vi "STP_Engine_Main.vi"(6 "Log Data?":bool, 8 "error in":errorcluster, 9 "notifier in":refnum<notifier>, 10 "Socket No":i16, 11 "Selected Sockets":i16[](array[numeric])) -> (0 "error out":errorcluster)   [LabVIEW 2023, in "HardwareAbstractionLayer_LVOOP.lvlib" / "CAN Application Protocols Lib.lvlib" / "STP Protocol.lvclass"]
uses:
  STP Protocol.lvclass
  Ctrls/STP Output Data.ctl
  Ctrls/STP Error Cluster.ctl
  Teststand Steptypes/CAN/CAN Engine/Control/CAN FGV State.ctl
  <vilib>/xnet/xnet.llb/XNET Frame CAN.ctl
  <vilib>/xnet/xnet.llb/XNET Frame Type CAN.ctl
  Ctrls/STP States.ctl
  Ctrls/STP Engine States.ctl
  Teststand Steptypes/CAN/CAN Engine/STP Engine SubVI/Control/STP Engine Rx Data.ctl
  Ctrls/STP Loop Data.ctl
  STP Protocol.lvclass/STP Protocol.ctl
  Ctrls/TP Frame Type.ctl
  0913cad6-f2c8-4594-8002-bcfba81b39ef.vi
  d64f42c0-1e64-4e1b-9106-5438a7ab598d.vi
  ddd6aa9f-f484-4e89-88b8-35a021554d50.vi
  7032564a-a6a9-40e0-a5d6-1f35f757e68a.vi
  Teststand Steptypes/LTT_TeststandSteptypes.lvlib
panel:
  out "RequestTimeout?":bool
  out "STP Output Data":T1
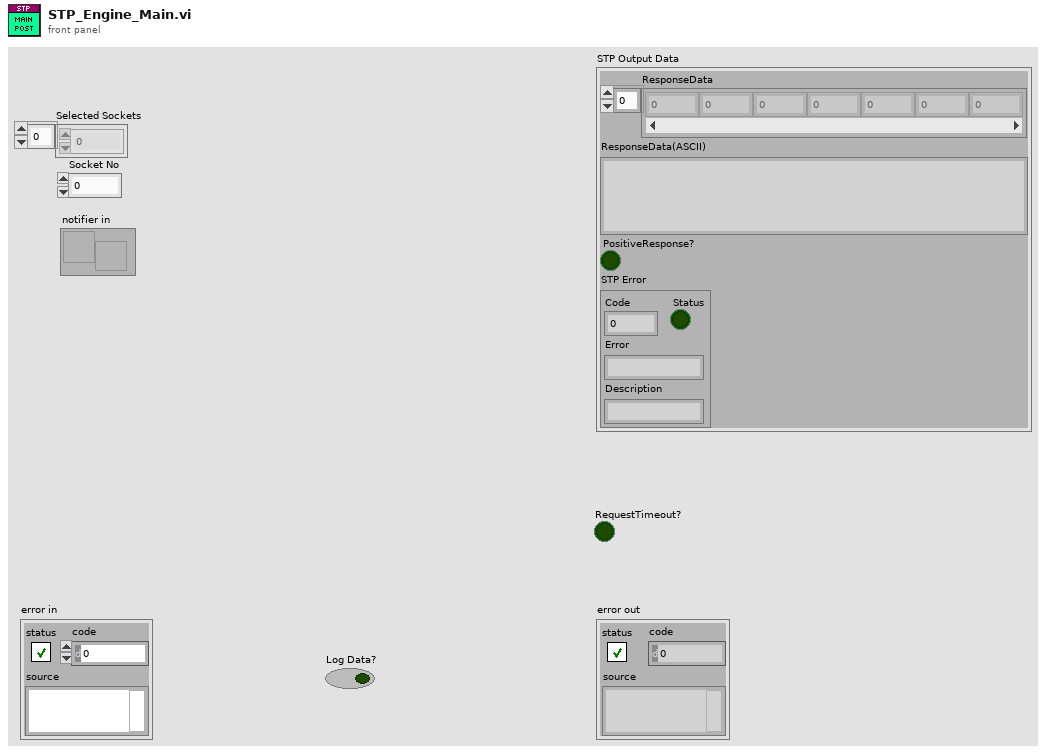
[diagram p1: front panel]
types:
  T1 = typedef "HardwareAbstractionLayer_LVOOP.lvlib/CAN Application Protocols Lib.lvlib/STP Protocol.lvclass/STP Output Data.ctl" = cluster{"ResponseData":u8[], "ResponseData(ASCII)":string, "PositiveResponse?":bool, "STP Error":T2}
  T2 = typedef "HardwareAbstractionLayer_LVOOP.lvlib/CAN Application Protocols Lib.lvlib/STP Protocol.lvclass/STP Error Cluster.ctl" = cluster{"Status":bool, "Code":u8, "Error":string, "Description":string}
  T3 = typedef "XNET Frame CAN.ctl" = cluster{"timestamp":timestamp, "payload":u8[], "identifier":u32, "type":T4, "extended?":bool, "echo?":bool}
  T4 = typedef "XNET Frame Type CAN.ctl" = u8
  T5 = typedef "LTT_TeststandSteptypes.lvlib/CAN FGV State.ctl" = enum16{"Init", "Get", "Set"}
  T6 = typedef "HardwareAbstractionLayer_LVOOP.lvlib/CAN Application Protocols Lib.lvlib/STP Protocol.lvclass/STP Engine States.ctl" = enum16{"Idle", "Poll", "Run"}
  T7 = typedef "HardwareAbstractionLayer_LVOOP.lvlib/CAN Application Protocols Lib.lvlib/STP Protocol.lvclass/STP States.ctl" = enum16{"Init", "Send Request", "Check Ack", "Send TP Frames", "Send Flow Control Frame", "Check Response", "Read TP Data", "Return Data", "Return Positive Response", "Return Error Response", "Exit"}
  T8 = typedef "LTT_TeststandSteptypes.lvlib/STP Engine Rx Data.ctl" = cluster{"STP Output Data":T1, "RequestTimeout?":bool}
  T9 = typedef "HardwareAbstractionLayer_LVOOP.lvlib/CAN Application Protocols Lib.lvlib/STP Protocol.lvclass/STP Loop Data.ctl" = cluster{"ResponseData":u8[], "DataSize(bytes)":u16, "ReceiveAllData?":bool, "PositiveResponse?":bool, "CosecutiveFrameID":fxp<+,4,4>, "#FrameToRead":i32}
  T10 = typedef "LTT_TeststandSteptypes.lvlib/STP Engine Tx Data.ctl" = cluster{"STP Input Data":T11, "Socket No":u16}
  T11 = typedef "HardwareAbstractionLayer_LVOOP.lvlib/CAN Application Protocols Lib.lvlib/STP Protocol.lvclass/STP Input Data.ctl" = cluster{"TxID":u32, "RxID":u32, "CMD":T12, "RQ Data":u8[], "+veResponseCode":u8, "ResponseTimeout (S)":dbl}
  T12 = typedef "HardwareAbstractionLayer_LVOOP.lvlib/CAN Application Protocols Lib.lvlib/STP Protocol.lvclass/STP CMD.ctl" = u8
  T13 = typedef "HardwareAbstractionLayer_LVOOP.lvlib/CAN Application Protocols Lib.lvlib/STP Protocol.lvclass/TP Frame Type.ctl" = u8
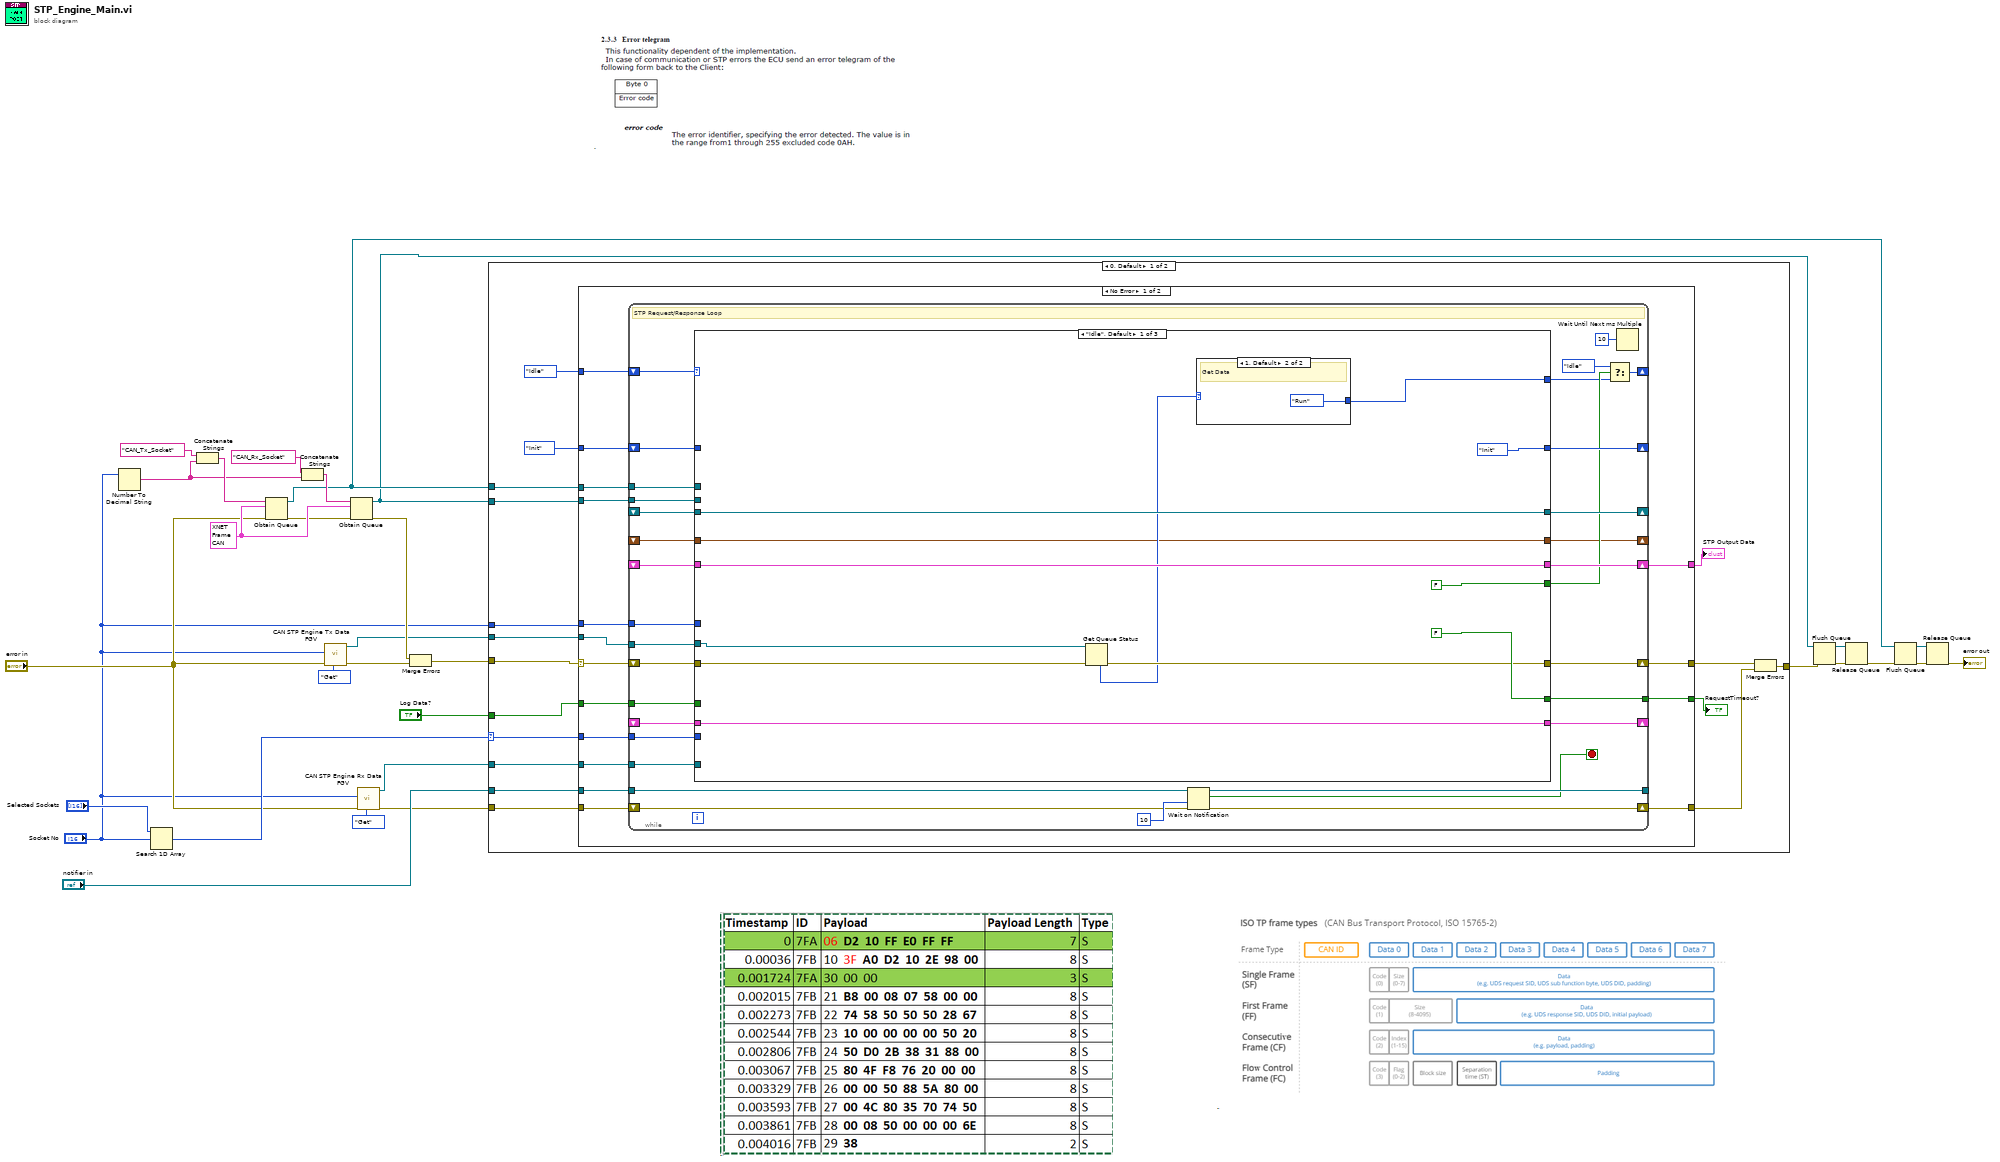
[diagram p0: block diagram]
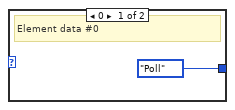
[diagram p2: hidden frame]
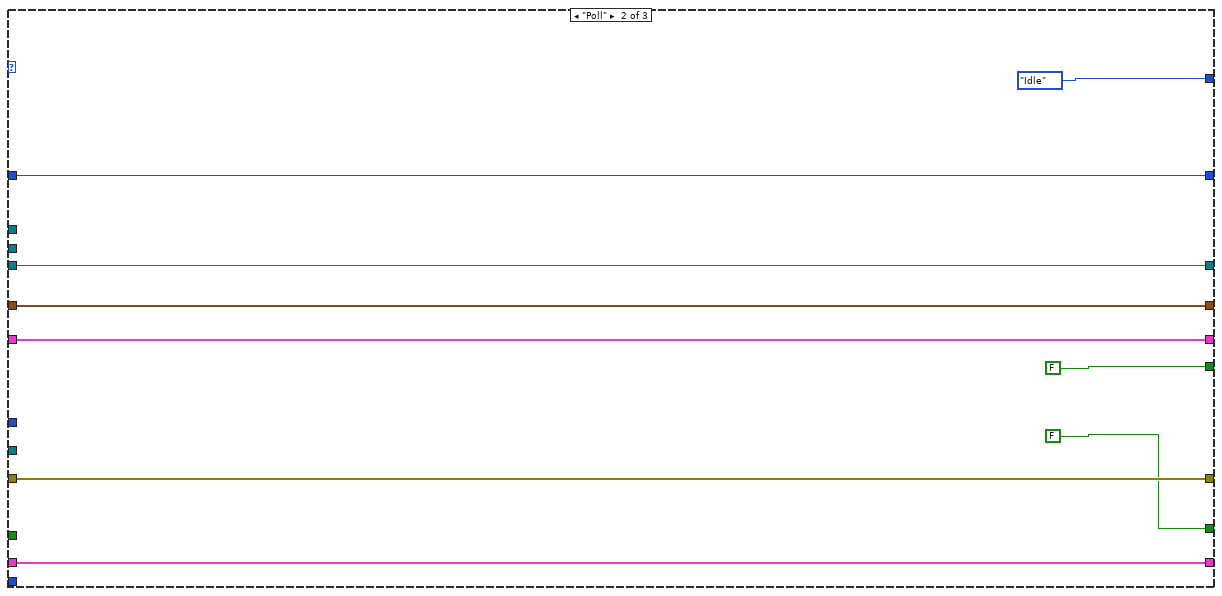
[diagram p3: hidden frame]
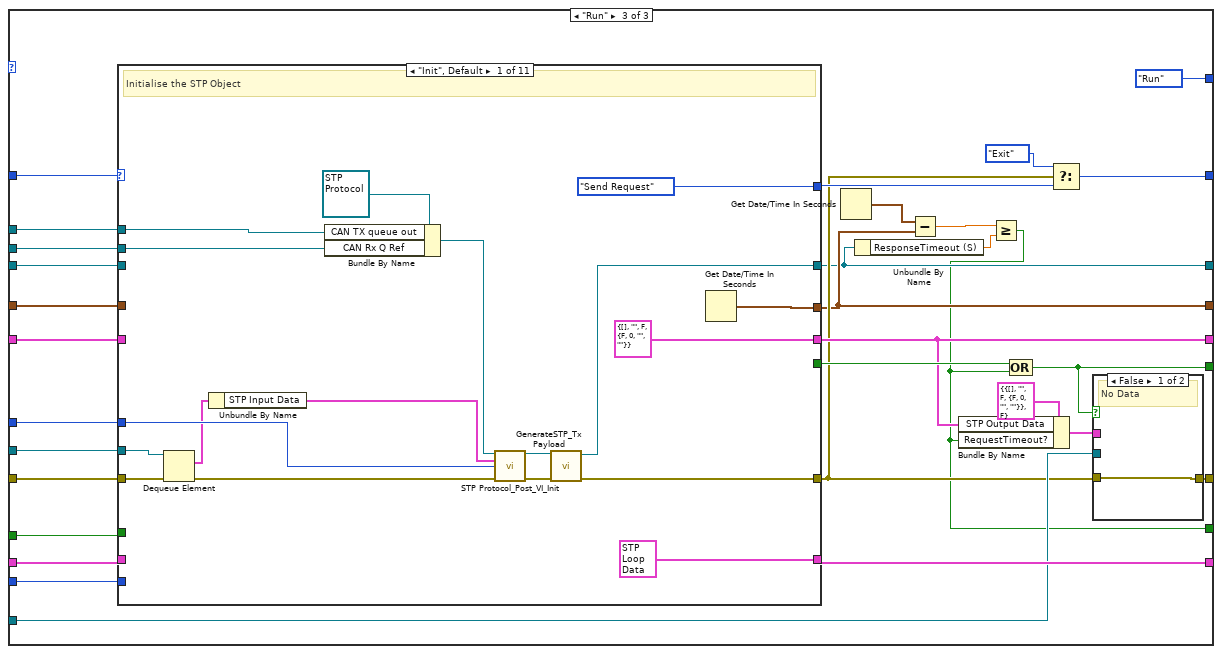
[diagram p4: hidden frame]
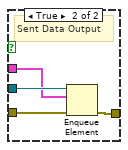
[diagram p5: hidden frame]
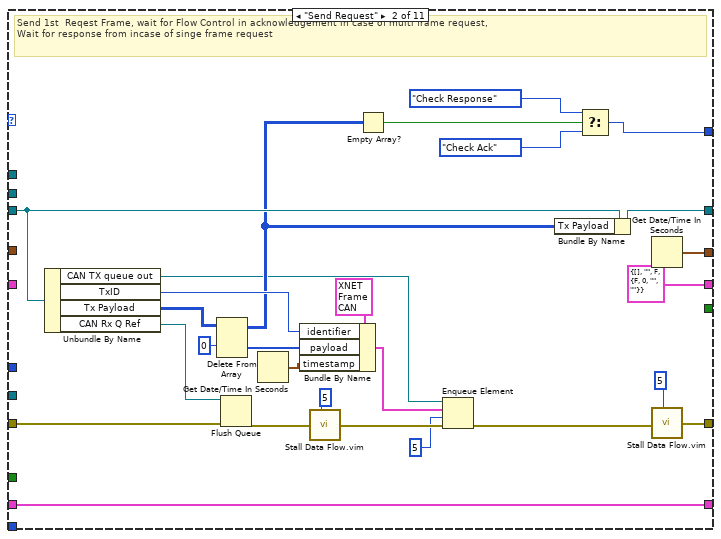
[diagram p6: hidden frame]
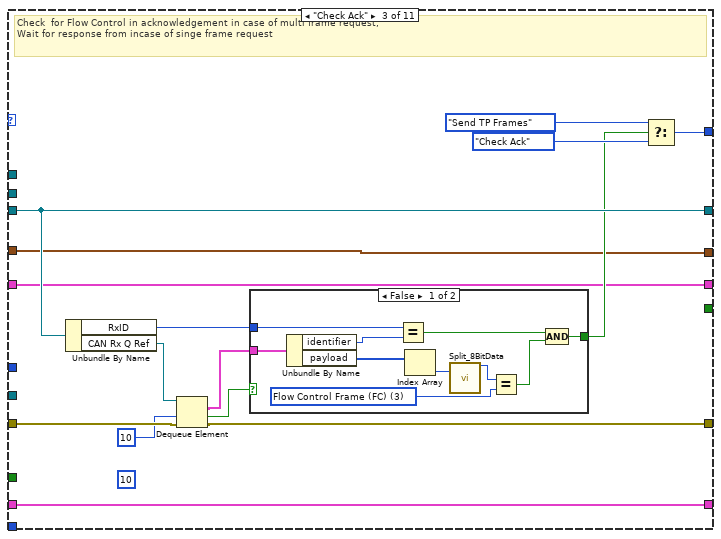
[diagram p7: hidden frame]
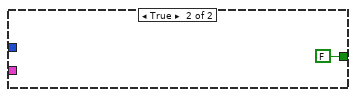
[diagram p8: hidden frame]
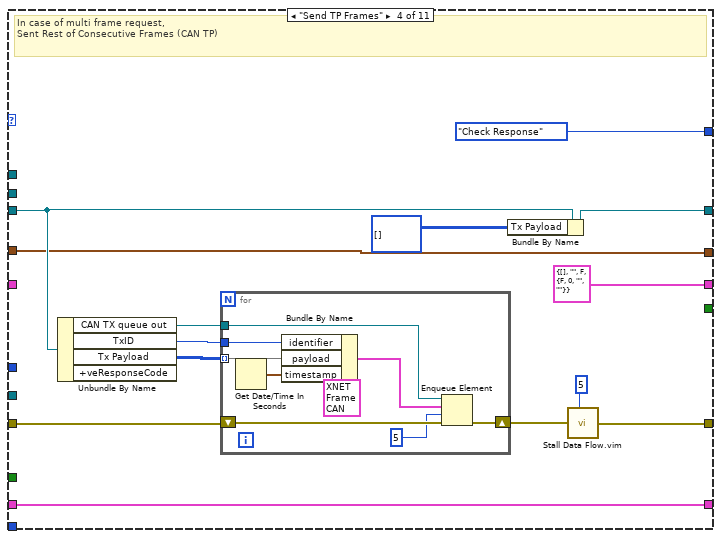
[diagram p9: hidden frame]
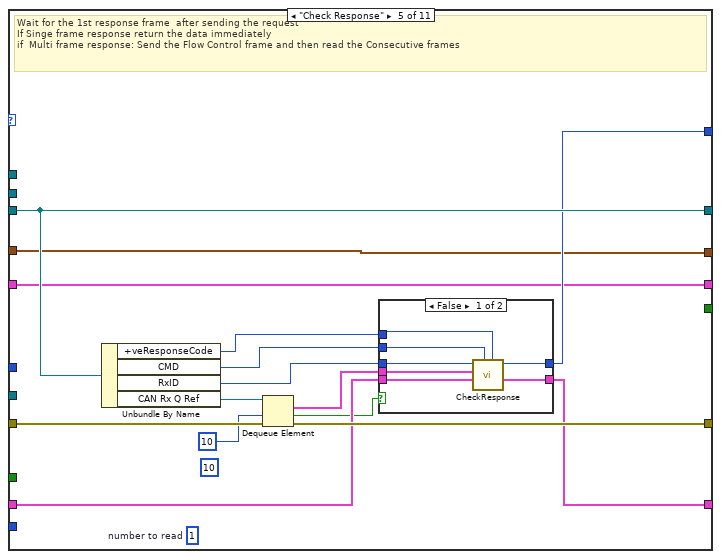
[diagram p10: hidden frame]
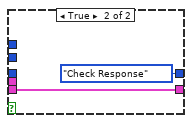
[diagram p11: hidden frame]
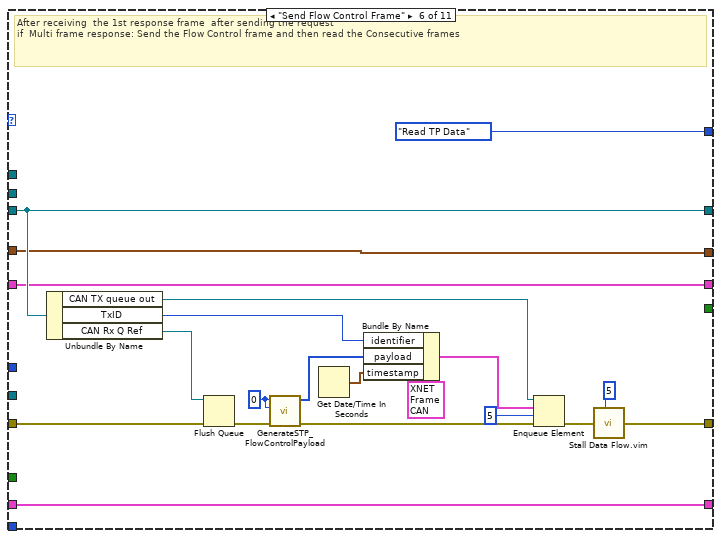
[diagram p12: hidden frame]
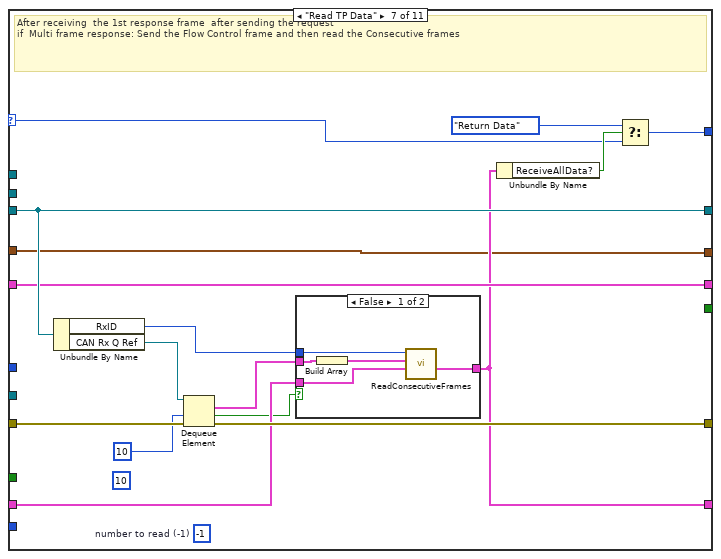
[diagram p13: hidden frame]
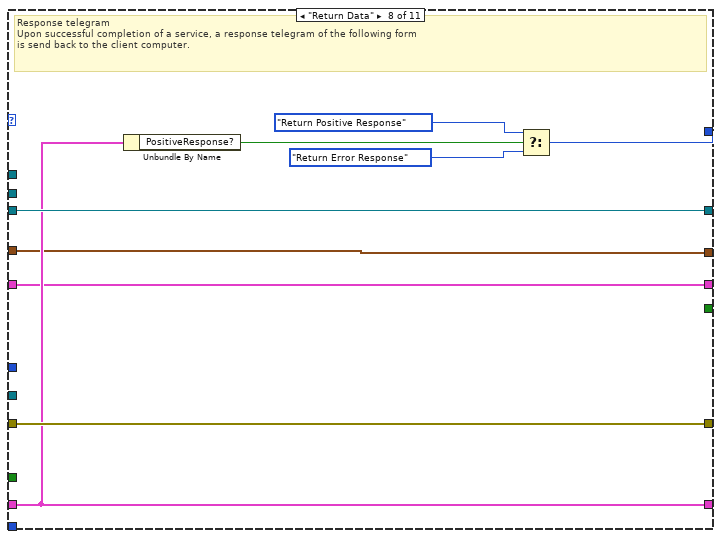
[diagram p15: hidden frame]
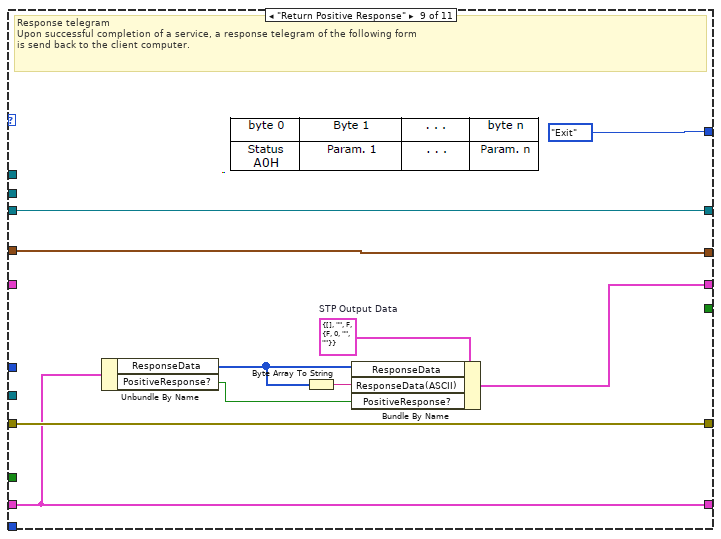
[diagram p16: hidden frame]
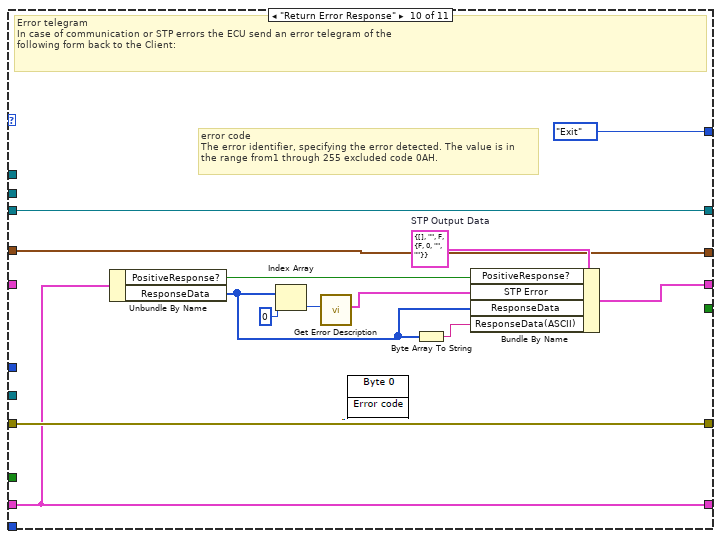
[diagram p17: hidden frame]
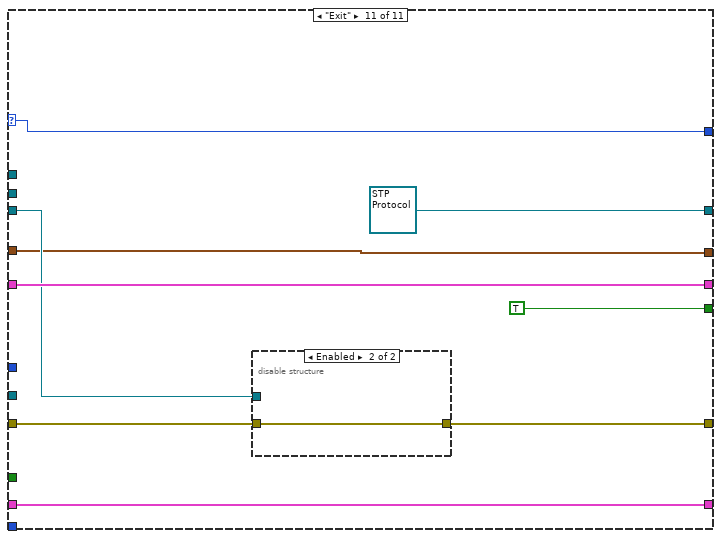
[diagram p18: hidden frame]
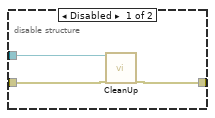
[diagram p19: hidden frame]
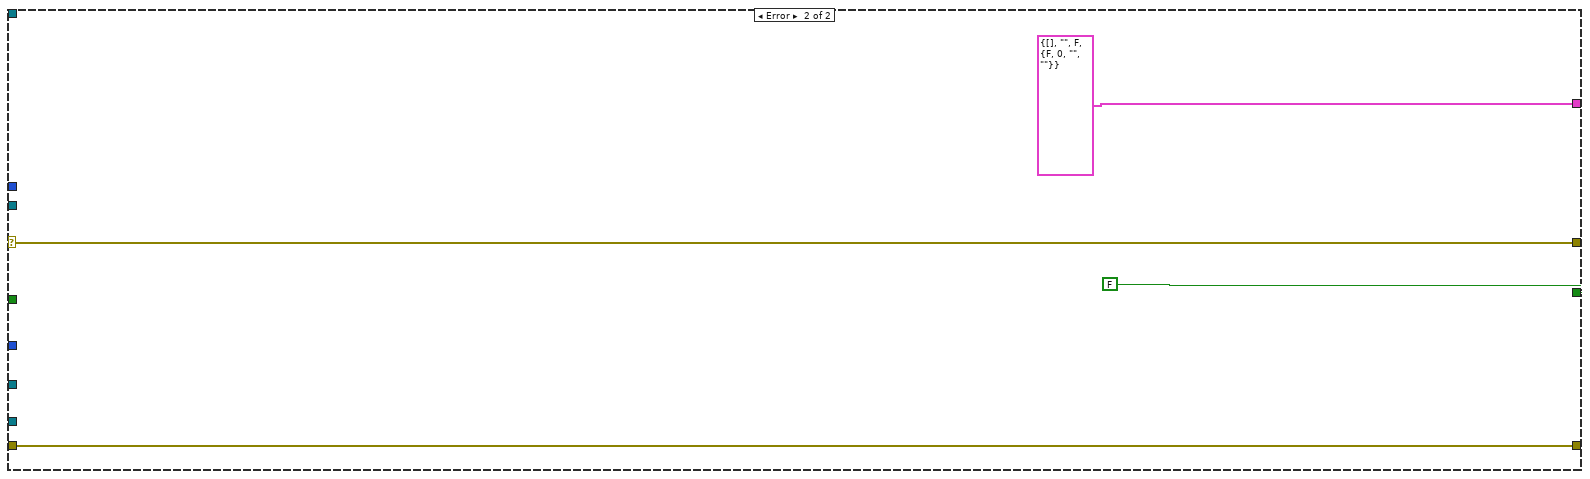
[diagram p20: hidden frame]
diagram:
  w16 = T3 {"timestamp"=timestamp(0 s since 1904-01-01), "payload"=[], "identifier"=0, "type"=0, "extended?"=FALSE, "echo?"=FALSE} ("CAN frame")
  n1 = Number To Decimal String(number="Socket No") -> (decimal integer string=w14:string)  [unwired: 1 in]
  n2 = Search 1D Array(1D array="Selected Sockets", element="Socket No") -> (index of element=w29:i32)  [unwired: 1 in]
  n3 = Concatenate Strings("CAN_Tx_Socket" ("name (unnamed)"), w14) -> (w20:string)
  n4 = Obtain Queue(name (unnamed)=w20, element data type=w16, error in (no error)="error in") -> (queue out=w6:refnum<queue>, error out=w15:errorcluster)  [unwired: 2 in, 1 out]
  n5 = Concatenate Strings("CAN_Rx_Socket" ("name (unnamed)"), w14) -> (w18:string)
  n6 = call "CAN STP Engine Tx Data FGV.vi"("CAN FGV State"=CAN_FGV_State."Get", "error in"="error in", "Socket No"="Socket No") -> ("error out"=w24:errorcluster, "STP Engine Tx Data out"=w3:refnum<queue>)  [unwired: 6 in, 1 out]
  n7 = Obtain Queue(name (unnamed)=w18, element data type=w16, error in (no error)=w15) -> (queue out=w5:refnum<queue>, error out=w12:errorcluster)  [unwired: 2 in, 1 out]
  n8 = call "CAN STP Engine Rx Data FGV.vi"("CAN FGV State"=CAN_FGV_State."Get", "error in"="error in", "Socket No"="Socket No") -> ("error out"=w22:errorcluster, "STP Engine Rx Data Out"=w4:refnum<queue>)  [unwired: 7 in]
  n9 = Merge Errors(w12, w24) -> (w13:errorcluster)
  n10 = case shown="0, Default" w29 {
    selector: w29 -> [w34 _]
    tunnel: "notifier in" -> [w47 _]
    tunnel: "Log Data?" -> [w43 _]
    tunnel: [w39 w364] -> w25
    tunnel: w3 -> [w38 _]
    tunnel: "Socket No" -> [w37 _]
    tunnel: w22 -> [w36 _]
    tunnel: w4 -> [w35 _]
    tunnel: w13 -> [w33 w364]
    tunnel: w6 -> [w32 _]
    tunnel: w5 -> [w31 _]
    frame 0, Default {
      n11 = case shown="No Error" w33 {
        selector: w33 -> [w62 w363]
        tunnel: [w63 w363] -> w41
        tunnel: STP_States."Init" -> [w61 _]
        tunnel: [w60 T1 {"ResponseData"=[], "ResponseData(ASCII)"="", "PositiveResponse?"=FALSE, "STP Error"={"Status"=FALSE, "Code"=0, "Error"="", "Description"=""}} ("STP Output Data")] -> w45
        tunnel: [w59 FALSE ("TimeLapsed?")] -> w44
        tunnel: w43 -> [w58 _]
        tunnel: w37 -> [w57 _]
        tunnel: STP_Engine_States."Idle" ("STP Engine States") -> [w56 _]
        tunnel: w47 -> [w55 _]
        tunnel: w36 -> [w54 w360]
        tunnel: [w51 w360] -> w40
        tunnel: w38 -> [w53 _]
        tunnel: w35 -> [w52 _]
        tunnel: w34 -> [w50 _]
        tunnel: w32 -> [w48 _]
        tunnel: w31 -> [w49 _]
        frame No Error {
          n12 = while {
            shift-right: [w83] -> _
            shift-left: _ -> [w95]
            shift-right: [w86] -> _
            shift-left: w61 -> [w94]
            shift-right: [w91] -> _
            shift-left: _ -> [w90]
            tunnel: [w82] -> w59
            shift-right: [w89] -> w60
            shift-left: _ -> [w88]
            tunnel: w58 -> [w87]
            tunnel: w57 -> [w85]
            shift-right: [w92] -> w63
            shift-left: w62 -> [w93]
            shift-right: [w73] -> _
            shift-left: w56 -> [w81]
            tunnel: w55 -> [w77]
            tunnel: [w75] -> _
            tunnel: w53 -> [w74]
            tunnel: w52 -> [w72]
            shift-right: [w69] -> w51
            shift-left: w54 -> [w76]
            tunnel: w50 -> [w68]
            shift-right: [w67] -> _
            shift-left: _ -> [w66]
            tunnel: w49 -> [w65]
            tunnel: w48 -> [w64]
            stop <- w71 stop-if-true
            # "STP Request/Response Loop"
            n13 = case shown="\"Idle\", Default" w81 {
              tunnel: w95 -> [w107 w116 w124]
              tunnel: w94 -> [_ w117 w149]
              tunnel: w93 -> [w102 w114 w148]
              tunnel: [FALSE FALSE w134] -> w80
              tunnel: [w101 w114 w136] -> w92
              tunnel: [w105 w113 w147] -> w91
              tunnel: w90 -> [w105 w113 w146]
              tunnel: [w106 w115 w132] -> w89
              tunnel: w88 -> [w106 w115 w145]
              tunnel: w87 -> [_ _ w144]
              tunnel: [STP_States."Init" w117 w142] -> w86
              tunnel: w85 -> [_ _ w140]
              tunnel: [w107 w116 w123] -> w83
              tunnel: [FALSE ("TimeLapsed?") FALSE ("TimeLapsed?") w121] -> w82
              tunnel: [w98 STP_Engine_States."Idle" ("STP Engine States") STP_Engine_States."Run" ("STP Engine States")] -> w79
              tunnel: w74 -> [w100 _ w137]
              tunnel: w72 -> [_ _ w135]
              tunnel: w68 -> [_ _ w129]
              tunnel: [w96 w110 w126] -> w67
              tunnel: w66 -> [w96 w110 w128]
              tunnel: w65 -> [_ _ w120]
              tunnel: w64 -> [_ _ w119]
              frame "Idle", Default {
                n14 = Get Queue Status(queue=w100, error in (no error)=w102) -> (error out=w101:errorcluster, # elements in queue=w99:i32)  [unwired: 1 in, 6 out]
                n15 = case shown="1, Default" w99 {
                  tunnel: [STP_Engine_States."Poll" ("STP Engine States") STP_Engine_States."Run" ("STP Engine States")] -> w98
                  frame 0 {
                    # "Element data #0"
                  }
                  frame 1, Default {
                    # "Get Data"
                  }
                }
              }
              frame "Poll" {
              }
              frame "Run" {
                n16 = case shown="\"Init\", Default" w149 {
                  selector: w149 -> [_ _ _ _ _ _ w302 _ _ _ w352]
                  tunnel: [w167 w193 w214 w237 w263 w292 w308 w323 w333 w346 refnum<class "STP Protocol.lvclass"> refnum ("STP Protocol out")] -> w123
                  tunnel: w124 -> [_ w199 w214 w239 w263 w292 w308 w323 w333 w346 w349]
                  tunnel: [w168 w183 w203 w231 w261 w281 w306 w322 w332 w345 w348] -> w130
                  tunnel: w148 -> [w163 w184 w205 w229 w262 w283 w307 w322 w332 w345 w350]
                  tunnel: [STP_States."Send Request" w188 w211 STP_States."Check Response" w257 STP_States."Read TP Data" w300 w319 STP_States."Exit" STP_States."Exit" w352] -> w143
                  tunnel: [T9 {"ResponseData"=[], "DataSize(bytes)"=0, "ReceiveAllData?"=FALSE, "PositiveResponse?"=FALSE, "CosecutiveFrameID"=1.0, "#FrameToRead"=0} ("STP Loop Data Out") w187 w208 w233 w252 w288 w298 w317 w330 w343 w355] -> w147
                  tunnel: w146 -> [_ w187 w208 w233 w258 w288 w297 w317 w330 w343 w355]
                  tunnel: [_ _ _ _ _ _ _ _ _ _ TRUE] -> w139
                  tunnel: [T1 {"ResponseData"=[], "ResponseData(ASCII)"="", "PositiveResponse?"=FALSE, "STP Error"={"Status"=FALSE, "Code"=0, "Error"="", "Description"=""}} ("STP Output Data") T1 {"ResponseData"=[], "ResponseData(ASCII)"="", "PositiveResponse?"=FALSE, "STP Error"={"Status"=FALSE, "Code"=0, "Error"="", "Description"=""}} ("STP Output Data") w207 T1 {"ResponseData"=[], "ResponseData(ASCII)"="", "PositiveResponse?"=FALSE, "STP Error"={"Status"=FALSE, "Code"=0, "Error"="", "Description"=""}} ("STP Output Data") w251 w284 w299 w316 w327 w341 w351] -> w132
                  tunnel: w145 -> [_ _ w207 _ w251 w284 w299 w316 _ _ w351]
                  tunnel: w144 -> [_ _ _ _ _ _ _ _ _ _ _]
                  tunnel: w140 -> [w165 _ _ _ _ _ _ _ _ _ _]
                  tunnel: w137 -> [w164 _ _ _ _ _ _ _ _ _ _]
                  tunnel: w129 -> [_ _ _ _ _ _ _ _ _ _ _]
                  tunnel: [w159 w173 w200 w226 w249 w273 w293 w315 w324 w334 w347] -> w126
                  tunnel: w128 -> [_ _ w200 w226 w249 w273 w293 w315 w324 w334 w347]
                  tunnel: w120 -> [w157 _ _ _ _ _ _ _ _ _ _]
                  tunnel: w119 -> [w158 _ _ _ _ _ _ _ _ _ _]
                  frame "Init", Default {
                    # "Initialise the STP Object"
                    n17 = Dequeue Element(queue=w164, error in (no error)=w163) -> (element=w161:T10, error out=w162:errorcluster)  [unwired: 1 in, 2 out]
                    n18 = Unbundle By Name(w161) -> ("STP Input Data"=w160:T11)
                    n19 = Bundle By Name(cluster=refnum<class "STP Protocol.lvclass"> refnum ("STP Protocol in"), "CAN TX queue out"=w158, "CAN Rx Q Ref"=w157) -> (w155:refnum<class "STP Protocol.lvclass">)
                    n20 = call "STP Protocol_Post_VI_Init.vi"("object in"=w155, "Init Data"=w160, "Socket No"=w165, "error in (no error)"=w162) -> ("object out"=w172:refnum<class "STP Protocol.lvclass">, "error out"=w171:errorcluster)  [unwired: 10 in]
                    n21 = call "GenerateSTP_Tx Payload.vi"("error in (no error)"=w171, "STP Protocol in"=w172) -> ("error out"=w168:errorcluster, "STP Protocol out"=w167:refnum<class "STP Protocol.lvclass">)  [unwired: 8 in]
                    n22 = Get Date/Time In Seconds() -> (seconds since 1Jan1904=w159:timestamp)
                  }
                  frame "Send Request" {
                    # "Send 1st  Reqest Frame, wait for Flow Control in acknowledgement in case of multi frame request,\nWait for response from incase of singe frame request"
                    n23 = Unbundle By Name(w199) -> ("CAN TX queue out"=w181:refnum<queue>, "TxID"=w197:u32, "Tx Payload"=w196:u8[][], "CAN Rx Q Ref"=w185:refnum<queue>)
                    n24 = Delete From Array(array=w196, index (row)=0) -> (deleted portion=w194:u8[], array with subset deleted=w192:u8[][])  [unwired: 2 in]
                    n25 = Flush Queue(queue=w185, error in (no error)=w184) -> (error out=w179:errorcluster)  [unwired: 2 out]
                    n26 = Get Date/Time In Seconds() -> (seconds since 1Jan1904=w186:timestamp)
                    n27 = Bundle By Name(cluster=T3 {"timestamp"=timestamp(0 s since 1904-01-01), "payload"=[], "identifier"=0, "type"=0, "extended?"=FALSE, "echo?"=FALSE} ("CAN frame"), "identifier"=w197, "payload"=w194, "timestamp"=w186) -> (w180:T3)
                    n28 = call "Stall Data Flow.vim"("value in"=w179, "milliseconds to wait"=u32 5) -> ("value out"=w178:errorcluster)  [unwired: 1 out]
                    n29 = Empty Array?(array=w192) -> (empty?=w191:bool)
                    n30 = Enqueue Element(queue=w181, element=w180, timeout in ms (-1)=5, error in (no error)=w178) -> (error out=w174:errorcluster)  [unwired: 2 out]
                    n31 = Bundle By Name(cluster=w199, "Tx Payload"=w192) -> (w193:refnum<class "STP Protocol.lvclass">)
                    n32 = Select(t=STP_States."Check Response", s=w191, f=STP_States."Check Ack") -> (s? t:f=w188:T7)
                    n33 = Get Date/Time In Seconds() -> (seconds since 1Jan1904=w173:timestamp)
                    n34 = call "Stall Data Flow.vim"("value in"=w174, "milliseconds to wait"=u32 5) -> ("value out"=w183:errorcluster)  [unwired: 1 out]
                  }
                  frame "Check Ack" {
                    (unwired) 10 ("timeout in ms (-1)")
                    # "Check  for Flow Control in acknowledgement in case of multi frame request,\nWait for response from incase of singe frame request"
                    n35 = Unbundle By Name(w214) -> ("RxID"=w210:u32, "CAN Rx Q Ref"=w206:refnum<queue>)
                    n36 = Dequeue Element(queue=w206, timeout in ms (-1)=10, error in (no error)=w205) -> (element=w202:T3, timed out?=w201:bool, error out=w203:errorcluster)  [unwired: 1 out]
                    n37 = case shown="False" w201 {
                      tunnel: w210 -> [w223 _]
                      tunnel: [w217 FALSE] -> w209
                      tunnel: w202 -> [w216 _]
                      frame False {
                        w220 = T13 3 items=["Single Frame (SF)", "First Frame (SF)", "Consecutive Frame (CF)", "Flow Control Frame (FC)"] ("Ring")
                        n38 = Unbundle By Name(w216) -> ("identifier"=w224:u32, "payload"=w222:u8[])
                        n39 = Equal?(x=w223, y=w224) -> (x = y?=w219:bool)
                        n40 = Index Array(array=w222) -> (element=w221:u8)  [unwired: 1 in]
                        n41 = call "Split_8BitData.vi"("x"=w221) -> ("hi(x)"=w215:u8)  [unwired: 17 in, 1 out]
                        n42 = Equal?(x=w215, y=w220) -> (x = y?=w218:bool)
                        n43 = Compound Arithmetic op=AND(w219, w218) -> (w217:bool)
                      }
                      frame True {
                      }
                    }
                    n44 = Select(t=STP_States."Send TP Frames", s=w209, f=STP_States."Check Ack") -> (s? t:f=w211:T7)
                  }
                  frame "Send TP Frames" {
                    # "In case of multi frame request,\nSent Rest of Consecutive Frames (CAN TP)"
                    n45 = Unbundle By Name(w239) -> ("CAN TX queue out"=w228:refnum<queue>, "TxID"=w238:u32, "Tx Payload"=w234:u8[][])  [unwired: 1 out]
                    n46 = for {
                      tunnel: w238 -> [w248]
                      tunnel: w234 -> [w247] mode=indexing
                      tunnel: w228 -> [w244]
                      shift-right: [w241] -> w227
                      shift-left: w229 -> [w243]
                      n47 = Get Date/Time In Seconds() -> (seconds since 1Jan1904=w246:timestamp)
                      n48 = Bundle By Name(cluster=T3 {"timestamp"=timestamp(0 s since 1904-01-01), "payload"=[], "identifier"=0, "type"=0, "extended?"=FALSE, "echo?"=FALSE} ("CAN frame"), "identifier"=w248, "payload"=w247, "timestamp"=w246) -> (w240:T3)
                      n49 = Enqueue Element(queue=w244, element=w240, timeout in ms (-1)=5, error in (no error)=w243) -> (error out=w241:errorcluster)  [unwired: 2 out]
                    }
                    n50 = Bundle By Name(cluster=w239, "Tx Payload"=u8[][] []) -> (w237:refnum<class "STP Protocol.lvclass">)
                    n51 = call "Stall Data Flow.vim"("value in"=w227, "milliseconds to wait"=u32 5) -> ("value out"=w231:errorcluster)  [unwired: 1 out]
                  }
                  frame "Check Response" {
                    (unwired) 10 ("timeout in ms (-1)")
                    (unwired) 1  # number to read
                    # "Wait for the 1st response frame  after sending the request\nIf Singe frame response return the data immediately\nif  Multi frame response: Send the Flow Control frame and then read the Consecutive frames"
                    n52 = Unbundle By Name(w263) -> ("+veResponseCode"=w254:u8, "CMD"=w255:T12, "RxID"=w256:u32, "CAN Rx Q Ref"=w260:refnum<queue>)
                    n53 = Dequeue Element(queue=w260, timeout in ms (-1)=10, error in (no error)=w262) -> (element=w259:T3, timed out?=w250:bool, error out=w261:errorcluster)  [unwired: 1 out]
                    n54 = case shown="False" w250 {
                      tunnel: w259 -> [w270 _]
                      tunnel: w258 -> [w269 w272]
                      tunnel: [w268 STP_States."Check Response" ("STP_NextState")] -> w257
                      tunnel: w256 -> [w267 _]
                      tunnel: w255 -> [w266 _]
                      tunnel: w254 -> [w265 _]
                      tunnel: [w264 w272] -> w252
                      frame False {
                        n55 = call "CheckResponse.vi"("+veResponseCode"=w265, "STP CMD"=w266, "STP Loop Data In"=w269, "Rx CAN frame"=w270, "RxID"=w267) -> ("STP Loop Data Out"=w264:T9, "STP_NextState"=w268:T7)  [unwired: 4 in, 1 out]
                      }
                      frame True {
                      }
                    }
                  }
                  frame "Send Flow Control Frame" {
                    w287 = u8 0 ("BlockSize(BS)")
                    # "After receiving  the 1st response frame  after sending the request\nif  Multi frame response: Send the Flow Control frame and then read the Consecutive frames"
                    n56 = Unbundle By Name(w292) -> ("CAN TX queue out"=w278:refnum<queue>, "TxID"=w290:u32, "CAN Rx Q Ref"=w279:refnum<queue>)
                    n57 = Flush Queue(queue=w279, error in (no error)=w283) -> (error out=w280:errorcluster)  [unwired: 2 out]
                    n58 = call "GenerateSTP_FlowControlPayload.vi"("error in (no error)"=w280, "SeperationTime(ST)"=w287, "BlockSize(BS)"=w287) -> ("error out"=w275:errorcluster, "Flow Control Payload"=w286:u8[])  [unwired: 7 in]
                    n59 = Get Date/Time In Seconds() -> (seconds since 1Jan1904=w285:timestamp)
                    n60 = Bundle By Name(cluster=T3 {"timestamp"=timestamp(0 s since 1904-01-01), "payload"=[], "identifier"=0, "type"=0, "extended?"=FALSE, "echo?"=FALSE} ("CAN frame"), "identifier"=w290, "payload"=w286, "timestamp"=w285) -> (w277:T3)
                    n61 = Enqueue Element(queue=w278, element=w277, timeout in ms (-1)=5, error in (no error)=w275) -> (error out=w274:errorcluster)  [unwired: 2 out]
                    n62 = call "Stall Data Flow.vim"("value in"=w274, "milliseconds to wait"=u32 5) -> ("value out"=w281:errorcluster)  [unwired: 1 out]
                  }
                  frame "Read TP Data" {
                    (unwired) 10 ("timeout in ms (-1)")
                    (unwired) -1  # number to read (-1)
                    # "After receiving  the 1st response frame  after sending the request\nif  Multi frame response: Send the Flow Control frame and then read the Consecutive frames"
                    n63 = Unbundle By Name(w308) -> ("RxID"=w304:u32, "CAN Rx Q Ref"=w305:refnum<queue>)
                    n64 = Dequeue Element(queue=w305, timeout in ms (-1)=10, error in (no error)=w307) -> (element=w296:T3, timed out?=w294:bool, error out=w306:errorcluster)  [unwired: 1 out]
                    n65 = case shown="False" w294 {
                      tunnel: w304 -> [w313 _]
                      tunnel: [w312 w314] -> w298
                      tunnel: w297 -> [w311 w314]
                      tunnel: w296 -> [w310 _]
                      frame False {
                        n66 = Build Array(w310) -> (w309:T3[])
                        n67 = call "ReadConsecutiveFrames.vi"("STP Loop Data In"=w311, "CAN Data"=w309, "RxID"=w313) -> ("STP Loop Data Out"=w312:T9)  [unwired: 8 in]
                      }
                      frame True {
                      }
                    }
                    n68 = Unbundle By Name(w298) -> ("ReceiveAllData?"=w303:bool)
                    n69 = Select(t=STP_States."Return Data", s=w303, f=w302) -> (s? t:f=w300:T7)
                  }
                  frame "Return Data" {
                    # "Response telegram\nUpon successful completion of a service, a response telegram of the following form\nis send back to the client computer."
                    n70 = Unbundle By Name(w317) -> ("PositiveResponse?"=w321:bool)
                    n71 = Select(t=STP_States."Return Positive Response", s=w321, f=STP_States."Return Error Response") -> (s? t:f=w319:T7)
                  }
                  frame "Return Positive Response" {
                    w328 = T1 {"ResponseData"=[], "ResponseData(ASCII)"="", "PositiveResponse?"=FALSE, "STP Error"={"Status"=FALSE, "Code"=0, "Error"="", "Description"=""}}  # STP Output Data
                    # "Response telegram\nUpon successful completion of a service, a response telegram of the following form\nis send back to the client computer."
                    n72 = Unbundle By Name(w330) -> ("ResponseData"=w326:u8[], "PositiveResponse?"=w329:bool)
                    n73 = Byte Array To String(unsigned byte array=w326) -> (string=w325:string)
                    n74 = Bundle By Name(cluster=w328, "ResponseData"=w326, "ResponseData(ASCII)"=w325, "PositiveResponse?"=w329) -> (w327:T1)
                  }
                  frame "Return Error Response" {
                    w342 = T1 {"ResponseData"=[], "ResponseData(ASCII)"="", "PositiveResponse?"=FALSE, "STP Error"={"Status"=FALSE, "Code"=0, "Error"="", "Description"=""}}  # STP Output Data
                    # "error code\nThe error identifier, specifying the error detected. The value is in\nthe range from1 through 255 excluded code 0AH."
                    # "Error telegram\nIn case of communication or STP errors the ECU send an error telegram of the\nfollowing form back to the Client:"
                    n75 = Unbundle By Name(w343) -> ("PositiveResponse?"=w340:bool, "ResponseData"=w335:u8[])
                    n76 = Index Array(array=w335, index=0) -> (element=w338:u8)
                    n77 = call "Get Error Description.vi"("Code"=w338) -> ("STP Error"=w337:T2)  [unwired: 10 in]
                    n78 = Byte Array To String(unsigned byte array=w335) -> (string=w336:string)
                    n79 = Bundle By Name(cluster=w342, "PositiveResponse?"=w340, "STP Error"=w337, "ResponseData"=w335, "ResponseData(ASCII)"=w336) -> (w341:T1)
                  }
                  frame "Exit" {
                    n80 = disable-structure shown="Enabled" {
                      disable-tunnel: w350 -> [w358 w359]
                      disable-tunnel: w349 -> [w357 _]
                      disable-tunnel: [w356 w359] -> w348
                      frame Disabled {
                        n81 = call-dynamic "CleanUp.vi"("object in"=w357, "error in (no error)"=w358) -> ("error out"=w356:errorcluster)  [unwired: 16 in, 1 out]
                      }
                      frame Enabled {
                      }
                    }
                  }
                }
                n82 = Get Date/Time In Seconds() -> (seconds since 1Jan1904=w127:timestamp)
                n83 = Unbundle By Name(w123) -> ("ResponseTimeout (S)"=w122:dbl)
                n84 = Subtract(x=w127, y=w126) -> (x-y=w125:dbl)
                n85 = Greater Or Equal?(x=w125, y=w122) -> (x >= y?=w121:bool)
                n86 = Bundle By Name(cluster=T8 {"STP Output Data"={"ResponseData"=[], "ResponseData(ASCII)"="", "PositiveResponse?"=FALSE, "STP Error"={"Status"=FALSE, "Code"=0, "Error"="", "Description"=""}}, "RequestTimeout?"=FALSE} ("element"), "STP Output Data"=w132, "RequestTimeout?"=w121) -> (w131:T8)
                n87 = Compound Arithmetic op=OR(w139, w121) -> (w134:bool)
                n88 = Select(t=STP_States."Exit", s=w130, f=w143) -> (s? t:f=w142:T7)
                n89 = case shown="False" w134 {
                  tunnel: w130 -> [w150 w154]
                  tunnel: [w150 w153] -> w136
                  tunnel: w135 -> [_ w152]
                  tunnel: w131 -> [_ w151]
                  frame False {
                    # "No Data"
                  }
                  frame True {
                    # "Sent Data Output"
                    n90 = Enqueue Element(queue=w152, element=w151, error in (no error)=w154) -> (error out=w153:errorcluster)  [unwired: 1 in, 2 out]
                  }
                }
              }
            }
            n91 = Wait on Notification(notifier=w77, timeout in ms (-1)=10, error in (no error)=w76) -> (notifier out=w75:refnum<notifier>, notification=w71:bool, error out=w69:errorcluster)  [unwired: 1 in, 1 out]
            n92 = Select(t=STP_Engine_States."Idle", s=w80, f=w79) -> (s? t:f=w73:T6)
            n93 = Wait Until Next ms Multiple(millisecond multiple=u32 10) -> ()  [unwired: 1 out]
          }
        }
        frame Error {
        }
      }
      "STP Output Data" <- w45
      "RequestTimeout?" <- w44
      n94 = Merge Errors(w41, w40) -> (w39:errorcluster)
    }
    frame -1 {
    }
  }
  n95 = Flush Queue(queue=w5, error in (no error)=w25) -> (queue out=w10:refnum<queue>, error out=w11:errorcluster)  [unwired: 1 out]
  n96 = Release Queue(queue=w10, error in (no error)=w11) -> (error out=w7:errorcluster)  [unwired: 1 in, 2 out]
  n97 = Flush Queue(queue=w6, error in (no error)=w7) -> (queue out=w9:refnum<queue>, error out=w8:errorcluster)  [unwired: 1 out]
  n98 = Release Queue(queue=w9, error in (no error)=w8) -> (error out=→"error out":errorcluster)  [unwired: 1 in, 2 out]
